vi "Do-Fft-Fpga-Top-Level-Multiple-Lengths.vi"(8 "error in":errorcluster, 10 "FFT Size 2":u16(ring)=32 items=["16"=16, "32"=32], 11 "FFT Size 1":u16(ring)=16 items=["16"=16, "32"=32]) -> (0 "error out":errorcluster, 2 "Results Match! (2)":bool, 3 "Results Match! (1)":bool)   [LabVIEW 2014]
panel:
  out "Comparison failed at\nindex (2)":i32
  out "Expected Results 2":csg[](array[numeric])
  out "Results 2":csg[](array[numeric])
  out "Source 2":csg[](array[numeric])
  out "Results 1":csg[](array[numeric])
  out "Comparison failed at\nindex (1)":i32
  out "Expected Results 1":csg[](array[numeric])
  out "Source 1":csg[](array[numeric])
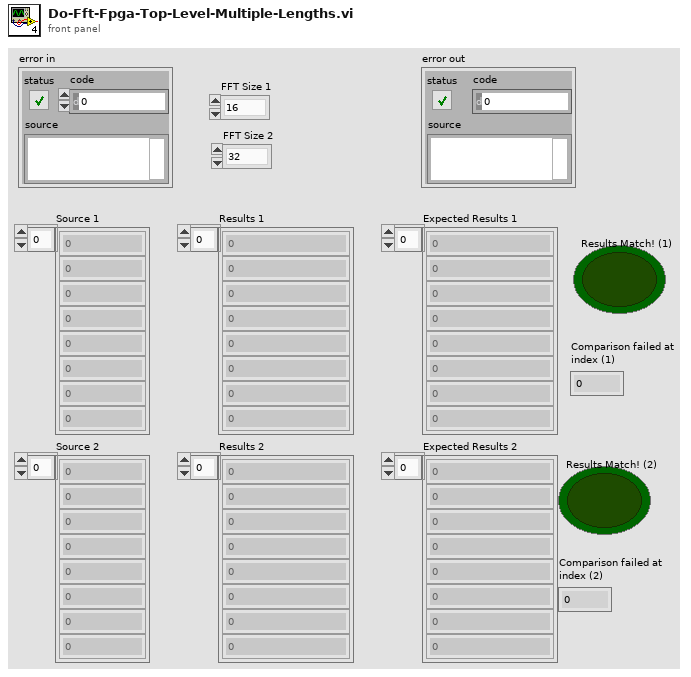
[diagram p1: front panel]
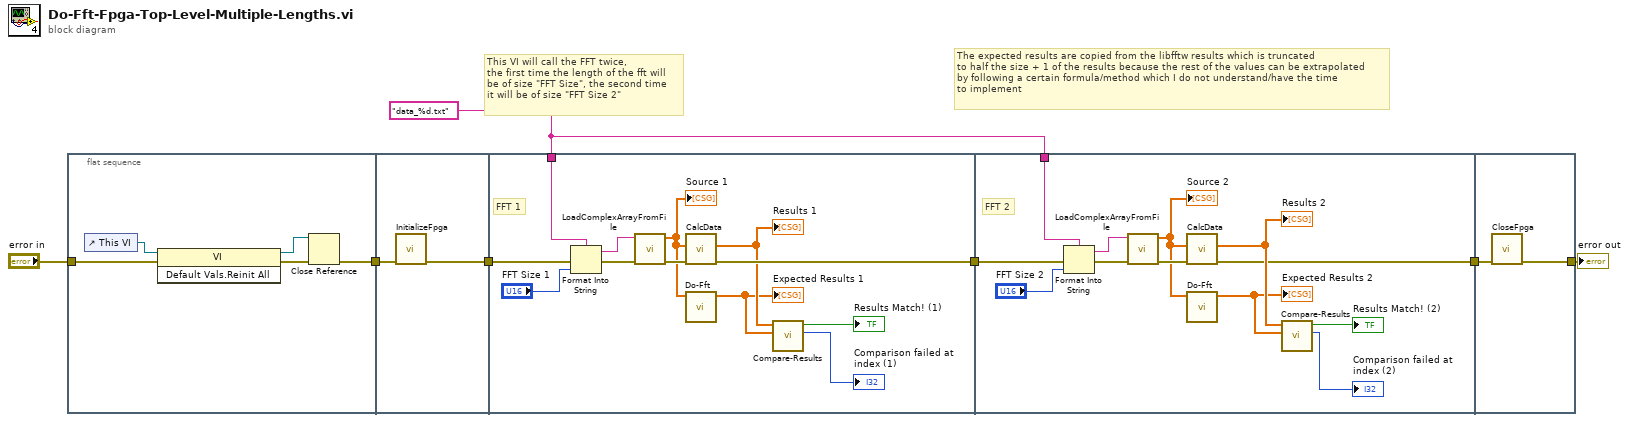
[diagram p0: block diagram]
diagram:
  w3 = "data_%d.txt"
  # "This VI will call the FFT twice,\nthe first time the length of the fft will\nbe of size \"FFT Size\", the second time\nit will be of size \"FFT Size 2\""
  # "The expected results are copied from the libfftw results which is truncated\nto half the size + 1 of the results because the rest of the values can be extrapolated\nby following a certain formula/method which I do not understand/have the time\nto implement"
  n1 = flat-sequence {
    tunnel: "error in" -> [w9]
    tunnel: [w8] -> w1
    tunnel: [w13] -> w7
    tunnel: w1 -> [w14]
    tunnel: w7 -> [w22]
    tunnel: [w26] -> w6
    tunnel: w3 -> [w15]
    tunnel: w6 -> [w35]
    tunnel: w3 -> [w33]
    tunnel: [w27] -> w2
    tunnel: [w40] -> w5
    tunnel: w2 -> [w39]
    frame #0 {
      n2 = control-ref of="This VI"() -> (w12:refnum<vi>)
      n3 = invoke class="VI" method="Default Vals.Reinit All"(reference=w12, error in=w9) -> (reference out=w10:refnum<vi>, error out=w11:errorcluster)  [unwired: 1 in, 1 out]
      n4 = Close Reference(reference=w10, error in (no error)=w11) -> (error out=w8:errorcluster)
    }
    frame #1 {
      n5 = call "InitializeFpga.vi"("error in"=w14) -> ("error out"=w13:errorcluster)  [unwired: 10 in]
    }
    frame #2 {
      # "FFT 1"
      n6 = Format Into String(format string=w15, error in=w22, "FFT Size 1") -> (resulting string=w24:string, error out=w25:errorcluster)  [unwired: 1 in]
      n7 = call "LoadComplexArrayFromFile.vi"("error in"=w25, "SourceFileName"=w24) -> ("error out"=w21:errorcluster, "Array"=w20:csg[])  [unwired: 8 in]
      "Source 1" <- w20
      n8 = call "CalcData.vi"("error in (no error)"=w21, "Complex Data (in)"=w20) -> ("error out"=w26:errorcluster, "Array out"=w19:csg[])  [unwired: 8 in]
      "Results 1" <- w19
      n9 = call "Do-Fft.vi"("X"=w20) -> ("FFT {X}"=w18:csg[])  [unwired: 10 in]
      "Expected Results 1" <- w18
      n10 = call "Compare-Results.vi"("FFT {X}"=w18, "Array in"=w19) -> ("Numeric"=→"Comparison failed at\nindex (1)":i32, "Boolean"=→"Results Match! (1)":bool)  [unwired: 8 in]
    }
    frame #3 {
      # "FFT 2"
      n11 = Format Into String(format string=w33, error in=w35, "FFT Size 2") -> (resulting string=w37:string, error out=w38:errorcluster)  [unwired: 1 in]
      n12 = call "LoadComplexArrayFromFile.vi"("error in"=w38, "SourceFileName"=w37) -> ("error out"=w36:errorcluster, "Array"=w32:csg[])  [unwired: 8 in]
      "Source 2" <- w32
      n13 = call "CalcData.vi"("error in (no error)"=w36, "Complex Data (in)"=w32) -> ("error out"=w27:errorcluster, "Array out"=w31:csg[])  [unwired: 8 in]
      "Results 2" <- w31
      n14 = call "Do-Fft.vi"("X"=w32) -> ("FFT {X}"=w30:csg[])  [unwired: 10 in]
      "Expected Results 2" <- w30
      n15 = call "Compare-Results.vi"("FFT {X}"=w30, "Array in"=w31) -> ("Numeric"=→"Comparison failed at\nindex (2)":i32, "Boolean"=→"Results Match! (2)":bool)  [unwired: 8 in]
    }
    frame #4 {
      n16 = call "CloseFpga.vi"("error in"=w39) -> ("error out"=w40:errorcluster)  [unwired: 10 in]
    }
  }
  "error out" <- w5
